vi "Edit Config.vi"(8 "error in (no error)":errorcluster, 11 "Single Query in":refnum<class "Single Query.lvclass">) -> (0 "error out":errorcluster, 3 "Single Query out":refnum<class "Single Query.lvclass">)   [LabVIEW 2024, in "Single Query.lvclass"]
doc: "Single Query.lvclass:Edit Config.vi\n\nThis VI is used to edit the Single Query configuration parameters.\n\nInstrument Communication Module Version 1.0\nDecember, 2017 Original Code Consulting David Thomson\n www.originalcode.com"
uses:
  Single Query.lvclass
  Single Query Config.ctl
  ICM Class Editor State.ctl
  ICM Editor Command.ctl
  Single Query.lvclass/Single Query.ctl
panel:
  in  "Flash Save":bool
  in  "Save":bool
  in  "Revert":bool
  in  "Single Query Config":T1
  # "The Single Query class is used for simple Query/Response\ninstruments, for which a single Query results in the instrument\nsending all the desired data channels."
  # "This parameter is displayed using the \"\\\" codes display.\nUse \\s for space, \\r for <CR>, \\n for <LF>, etc."
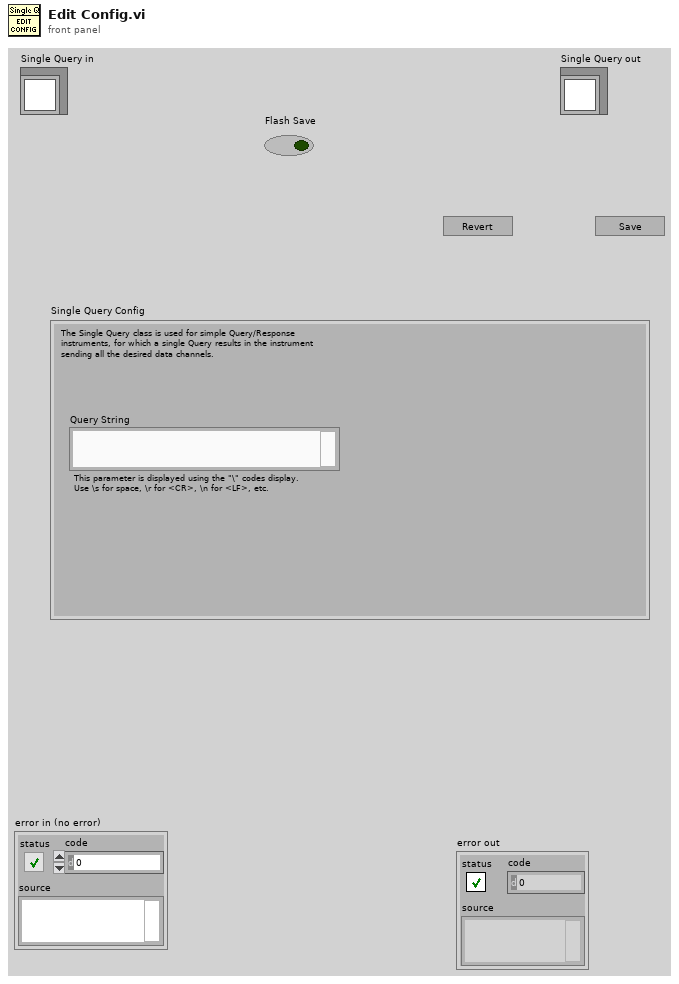
[diagram p1: front panel]
types:
  T1 = typedef "Single Query.lvclass/Single Query Config.ctl" = cluster{"Query String":string}
  T2 = typedef "ICM Editor Command.ctl" = enum16{"No-op", "Exit"}
  T3 = typedef "ICM Class Editor State.ctl" = enum16{"Init", "Wait", "Write", "Read", "Display", "Set Flashing", "Error", "Stop"}
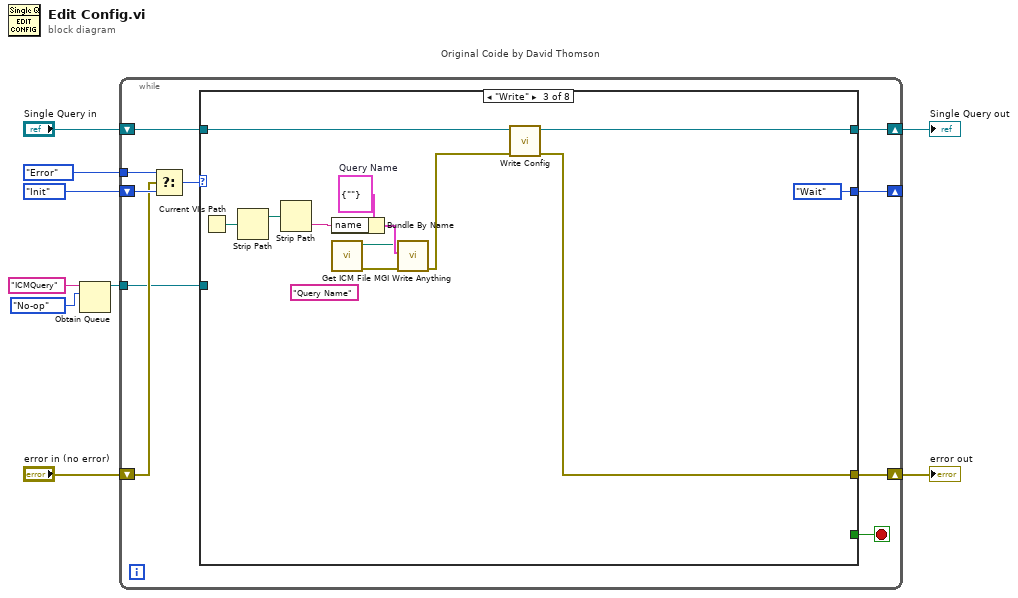
[diagram p0: block diagram]
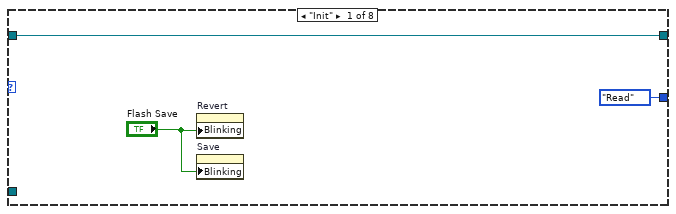
[diagram p2: hidden frame]
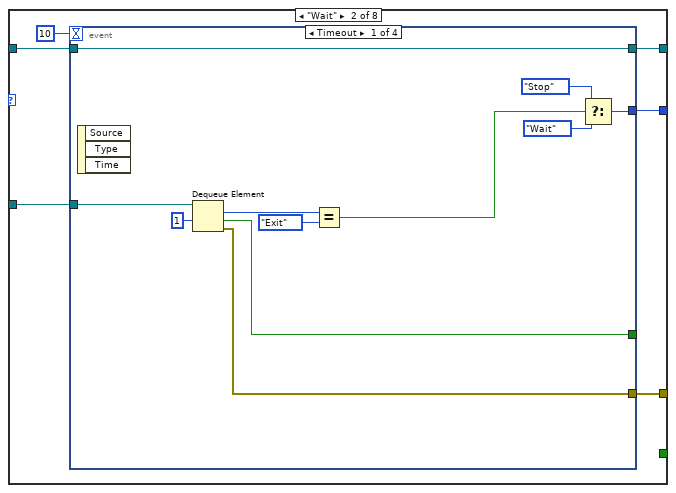
[diagram p3: hidden frame]
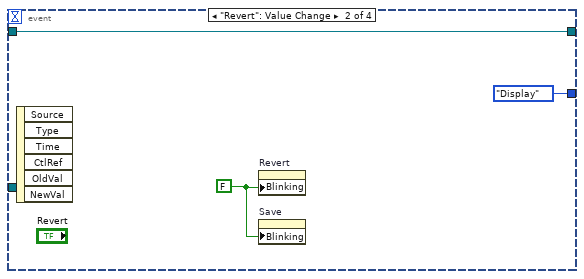
[diagram p4: hidden frame]
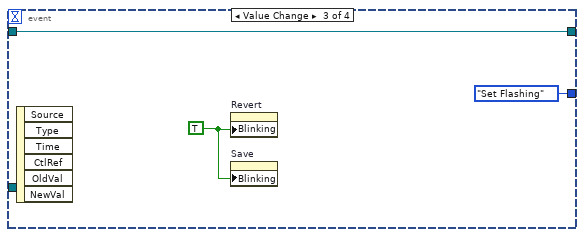
[diagram p5: hidden frame]
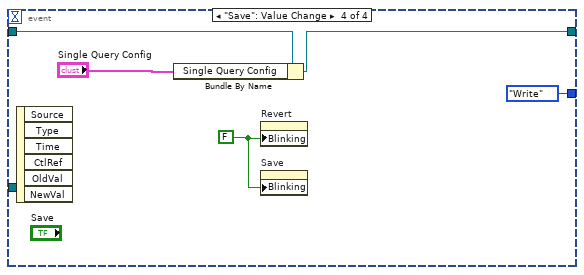
[diagram p6: hidden frame]
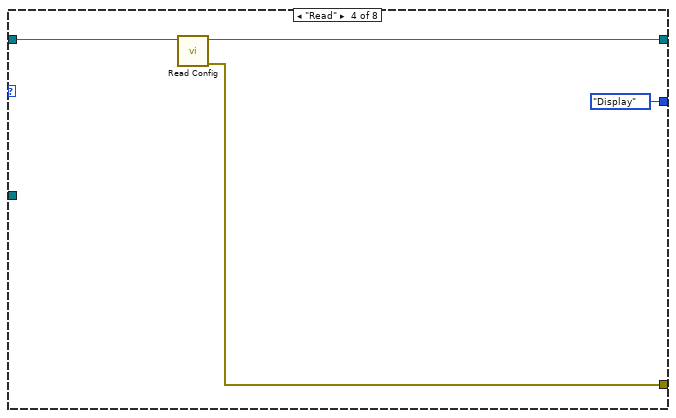
[diagram p7: hidden frame]
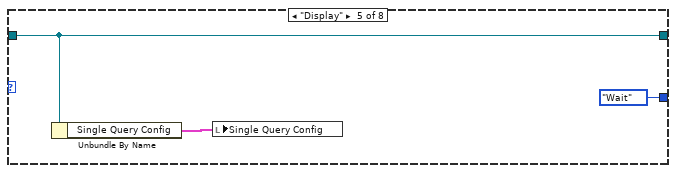
[diagram p8: hidden frame]
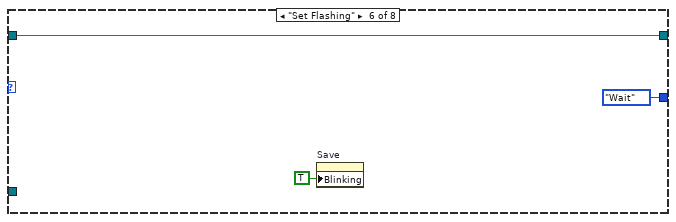
[diagram p9: hidden frame]
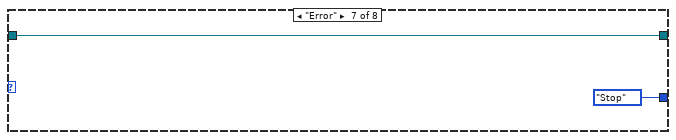
[diagram p10: hidden frame]
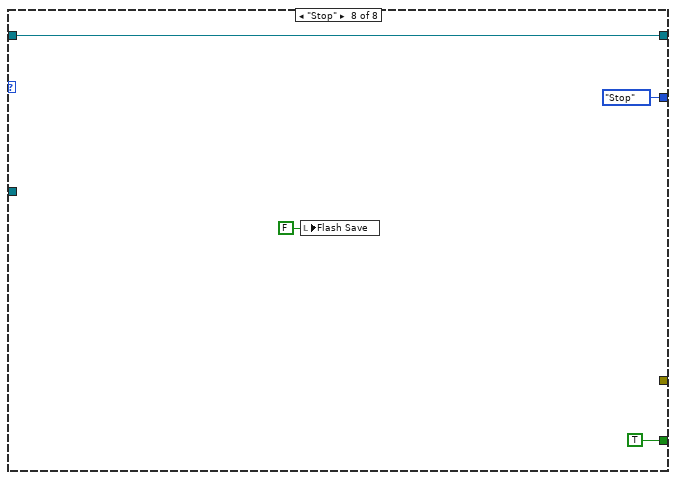
[diagram p11: hidden frame]
diagram:
  n1 = Obtain Queue(name (unnamed)="ICMQuery", element data type=ICM_Editor_Command."No-op" ("Editor Command")) -> (queue out=w1:refnum<queue>)  [unwired: 3 in, 2 out]
  n2 = while "Original Coide by David Thomson" {
    shift-right: [w19] -> w8
    shift-left: "Single Query in" -> [w18]
    shift-right: [w12] -> _
    shift-left: ICM_Class_Editor_State."Init" ("Config State") -> [w16]
    shift-right: [w11] -> w6
    shift-left: "error in (no error)" -> [w14]
    tunnel: ICM_Class_Editor_State."Error" ("Config State") -> [w13]
    tunnel: w1 -> [w10]
    stop <- w17 stop-if-true
    n3 = Select(t=w13, s=w14, f=w16) -> (s? t:f=w15:T3)
    n4 = case shown="\"Write\"" w15 {
      tunnel: [w21 w26 w60 w64 w69 w72 w74 w78] -> w19
      tunnel: w18 -> [w21 w25 w61 w66 w69 w72 w74 w78]
      tunnel: [_ _ _ _ _ _ _ TRUE] -> w17
      tunnel: [ICM_Class_Editor_State."Read" ("Config State") w27 ICM_Class_Editor_State."Wait" ("Config State") ICM_Class_Editor_State."Display" ("Config State") ICM_Class_Editor_State."Wait" ("Config State") ICM_Class_Editor_State."Wait" ("Config State") ICM_Class_Editor_State."Stop" ("Config State") ICM_Class_Editor_State."Stop" ("Config State")] -> w12
      tunnel: [_ w23 w59 w65 _ _ _ _] -> w11
      tunnel: w10 -> [_ w24 _ _ _ _ _ _]
      frame "Init" {
        n5 = property on="Revert" class="Bool"("Blinking"="Flash Save") -> ()  [unwired: 2 in, 2 out]
        n6 = property on="Save" class="Bool"("Blinking"="Flash Save") -> ()  [unwired: 2 in, 2 out]
      }
      frame "Wait" {
        n7 = event shown="[0] Timeout" {
          selector: _ -> [_ _ _ _]
          dyn-events: _ -> [_ _ _ _]
          timeout: 10 -> [_ _ _ _]
          tunnel: [w36 ICM_Class_Editor_State."Display" ("Config State") ICM_Class_Editor_State."Set Flashing" ("Config State") ICM_Class_Editor_State."Write" ("Config State")] -> w27
          tunnel: [w39 w41 w45 w47] -> w26
          tunnel: w25 -> [w39 w41 w45 w48]
          tunnel: w24 -> [w38 _ _ _]
          tunnel: [w30 _ _ _] -> w23
          tunnel: [w29 _ _ _] -> _
          event Timeout {
            n8 = event-data() -> ()  [unwired: 1 in, 3 out]
            n9 = Dequeue Element(queue=w38, timeout in ms (-1)=1) -> (element=w35:T2, timed out?=w29:bool, error out=w30:errorcluster)  [unwired: 1 in, 1 out]
            n10 = Equal?(x=w35, y=ICM_Editor_Command."Exit") -> (x = y?=w33:bool)
            n11 = Select(t=ICM_Class_Editor_State."Stop" ("Config State"), s=w33, f=ICM_Class_Editor_State."Wait" ("Config State")) -> (s? t:f=w36:T3)
          }
          event "Revert": Value Change {
            w40 = FALSE ("Blinking")
            n12 = event-data() -> ()  [unwired: 1 in, 6 out]
            n13 = property on="Revert" class="Bool"("Blinking"=w40) -> ()  [unwired: 2 in, 2 out]
            n14 = property on="Save" class="Bool"("Blinking"=w40) -> ()  [unwired: 2 in, 2 out]
          }
          event Value Change {
            w43 = TRUE ("Blinking")
            n15 = event-data() -> ()  [unwired: 1 in, 6 out]
            n16 = property on="Revert" class="Bool"("Blinking"=w43) -> ()  [unwired: 2 in, 2 out]
            n17 = property on="Save" class="Bool"("Blinking"=w43) -> ()  [unwired: 2 in, 2 out]
          }
          event "Save": Value Change {
            w46 = FALSE ("Blinking")
            n18 = event-data() -> ()  [unwired: 1 in, 6 out]
            n19 = Bundle By Name(cluster=w48, "Single Query Config"="Single Query Config") -> (w47:refnum<class "Single Query.lvclass">)
            n20 = property on="Revert" class="Bool"("Blinking"=w46) -> ()  [unwired: 2 in, 2 out]
            n21 = property on="Save" class="Bool"("Blinking"=w46) -> ()  [unwired: 2 in, 2 out]
          }
        }
      }
      frame "Write" {
        w55 = cluster{"name":string} {"name"=""}  # Query Name
        (unwired) "Query Name" ("Section Name (Name of \"Anything\")")
        n22 = Current VI's Path() -> (path=w58:path)
        n23 = Strip Path(path=w58) -> (stripped path=w57:path)  [unwired: 1 out]
        n24 = Strip Path(path=w57) -> (name=w54:string)  [unwired: 1 out]
        n25 = Bundle By Name(cluster=w55, "name"=w54) -> (w53:cluster{"name":string})
        n26 = call "Get ICM File.vi"() -> ("error out"=w56:errorcluster, "ICM File"=w51:path)  [unwired: 10 in]
        n27 = call "MGI Write Anything.vi"("Error In"=w56, "Anything"=w53, "Path (dialog)"=w51) -> ("Error Out"=w52:errorcluster)  [unwired: 6 in, 2 out]
        n28 = call-dynamic "Write Config.vi"("error in (no error)"=w52, "Single Query in"=w61) -> ("error out"=w59:errorcluster, "Single Query out"=w60:refnum<class "Single Query.lvclass">)  [unwired: 8 in]
      }
      frame "Read" {
        n29 = call-dynamic "Read Config.vi"("Single Query in"=w66) -> ("error out"=w65:errorcluster, "Single Query out"=w64:refnum<class "Single Query.lvclass">)  [unwired: 9 in]
      }
      frame "Display" {
        n30 = Unbundle By Name(w69) -> ("Single Query Config"=w68:T1)
        n31 = local write "Single Query Config"(w68) -> ()
      }
      frame "Set Flashing" {
        n32 = property on="Save" class="Bool"("Blinking"=TRUE) -> ()  [unwired: 2 in, 2 out]
      }
      frame "Error" {
      }
      frame "Stop" {
        n33 = local write "Flash Save"(FALSE ("Flash Save")) -> ()
      }
    }
  }
  "error out" <- w6
  "Single Query out" <- w8
